vi "AOTFStatus.vi"() -> ()   [LabVIEW 2013]
panel:
  in  "AOTF Status":string
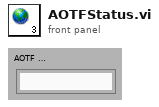
[diagram p1: front panel]
diagram:
